vi "Configure Storage Trace.vi"(0 "VISA resource name":refnum<visa-resource-name>, 5 "Storage Count (2)":i32=2 min=2 max=9999, 7 "Storage Mode (0:Off)":i32(ring) items=["Off", "Max Hold", "Average", "Min Hold", "Linear Average"], 11 "error in (no error)":errorcluster) -> (4 "VISA resource name out":refnum<visa-resource-name>, 15 "error out":errorcluster)   [LabVIEW 2020, in "Anritsu Signal Analyzer Series.lvlib"]
doc: "Configures the storage settings of the spectrum analyzer."
uses:
  Anritsu Signal Analyzer Series.lvlib
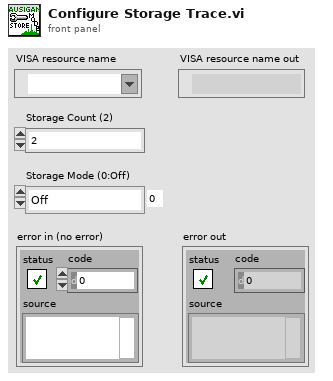
[diagram p1: front panel]
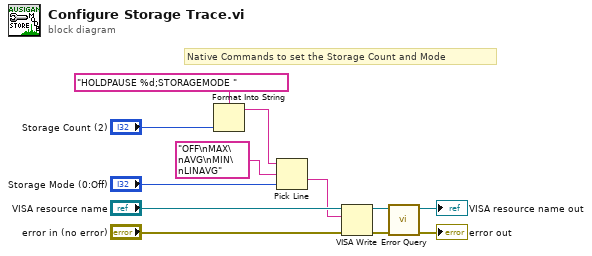
[diagram p0: block diagram]
diagram:
  # "Native Commands to set the Storage Count and Mode"
  n1 = Format Into String(format string="HOLDPAUSE %d;STORAGEMODE " ("Format String"), "Storage Count (2)") -> (resulting string=w2:string)  [unwired: 2 in, 1 out]
  n2 = Pick Line(string ("")=w2, multi-line string="OFF\nMAX\nAVG\nMIN\nLINAVG" ("_Case0"), line index="Storage Mode (0:Off)") -> (output string=w1:string)
  n3 = VISA Write(VISA resource name="VISA resource name", write buffer=w1, error in (no error)="error in (no error)") -> (VISA resource name out=w5:refnum<visa-resource-name>, error out=w6:errorcluster)  [unwired: 1 out]
  n4 = call "Error Query.vi"("error in (no error)"=w6, "VISA resource name"=w5) -> ("error out"=→"error out":errorcluster, "VISA resource name out"=→"VISA resource name out":refnum<visa-resource-name>)  [unwired: 6 in, 2 out]
